vi "TDMS Write.vi"(7 "Channel Name":string, 8 "error in (no error)":errorcluster, 9 "Group Name":string, 10 "TDMS in":refnum<k34>, 11 "Cluster in":refnum<class "Cluster.lvclass">) -> (0 "error out":errorcluster, 2 "TDMS Out":refnum<k34>)   [LabVIEW 2020, in "Data.lvlib" / "Cluster.lvclass"]
doc: "Write Generic Data to a TDMS file."
uses:
  Cluster.lvclass
  Cluster.lvclass/Cluster.ctl
  Generic Data.lvclass
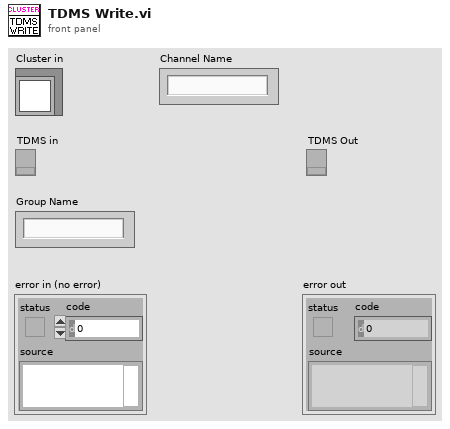
[diagram p1: front panel]
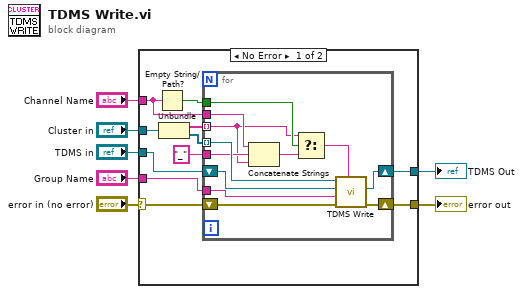
[diagram p0: block diagram]
diagram:
  n1 = case shown="No Error" "error in (no error)" {
    selector: "error in (no error)" -> [w13 w31]
    tunnel: [w12 w31] -> w1
    tunnel: "TDMS in" -> [w15 w32]
    tunnel: [w14 w32] -> w2
    tunnel: "Channel Name" -> [w9 _]
    tunnel: "Group Name" -> [w16 _]
    tunnel: "Cluster in" -> [w18 _]
    frame No Error {
      n2 = Empty String/Path?(string/path=w9) -> (empty?=w8:bool)
      n3 = Unbundle(w18) -> (w11:string[], w17:refnum<class "Generic Data.lvclass">[])
      n4 = for {
        tunnel: w17 -> [w30] mode=indexing
        tunnel: w16 -> [w29]
        shift-right: [w24] -> w14
        shift-left: w15 -> [w28]
        shift-right: [w23] -> w12
        shift-left: w13 -> [w27]
        tunnel: w9 -> [w26]
        tunnel: "_" ("string") -> [w25]
        tunnel: w11 -> [w21] mode=indexing
        tunnel: w8 -> [w22]
        n5 = Concatenate Strings(w26, w25, w21) -> (w20:string)
        n6 = Select(t=w21, s=w22, f=w20) -> (s? t:f=w19:string)
        n7 = call-dynamic "TDMS Write.vi"("Channel Name"=w19, "error in (no error)"=w27, "Group Name"=w29, "TDMS in"=w28, "Generic Data in"=w30) -> ("error out"=w23:errorcluster, "TDMS Out"=w24:refnum<k34>)  [unwired: 5 in]
      }
    }
    frame Error {
    }
  }
  "error out" <- w1
  "TDMS Out" <- w2
